vi "Add Rational Polynomials.vi"   [LabVIEW 2017, in "NI_AALPro.lvlib"]
doc: "Adds the rational polynomials G1 and G2. The data types you wire to the <B>Numerator 1</B>, <B>Denominator 1</B>, <B>Numerator 2</B>, and <B>Denominator 2</B> inputs determine the polymorphic instance to use."
uses:
  NI_AALPro.lvlib
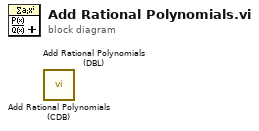
[diagram p0: block diagram]
diagram:
  n1 = call "Add Rational Polynomials (CDB).vi"() -> ()  [unwired: 9 in, 3 out]
  n2 = call "Add Rational Polynomials (DBL).vi"() -> ()  [unwired: 9 in, 3 out]
